vi "while_v0_v18.vi"() -> ()   [LabVIEW 2009]
panel:
  in  "Color Box":u32(colorbox)=16711695
  in  "X0":u16(slide)=73 scale=0.0..400.0
  in  "X1":u16(slide)=287 scale=0.0..400.0
  in  "Y1":u16(slide)=204 scale=300.0..0.0
  in  "Y0":u16(slide)=76 scale=300.0..0.0
  in  "stop":bool
  out "Picture":picture
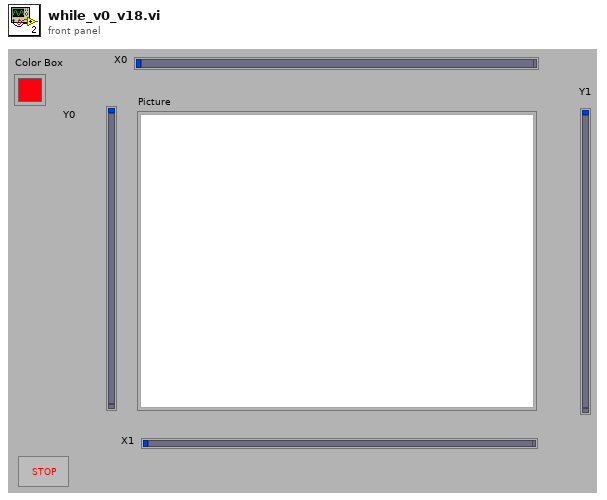
[diagram p1: front panel]
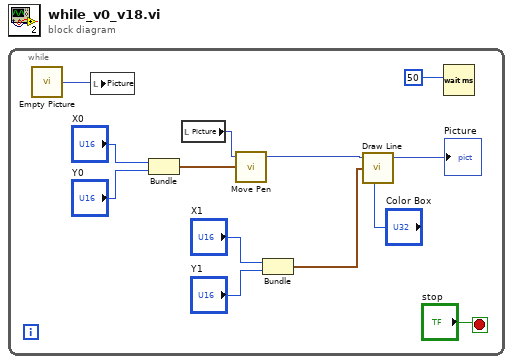
[diagram p0: block diagram]
diagram:
  n1 = while {
    stop <- "stop" stop-if-true
    n2 = call "Empty Picture"() -> ("empty picture"=w5:picture)
    n3 = local write "Picture"(w5) -> ()
    n4 = Bundle("X0"="X0", "Y0"="Y0") -> (w9:cluster{"X0":u16, "Y0":u16})  [unwired: 1 in]
    n5 = local read "Picture"() -> (w11:picture)
    n6 = call <vilib>:"Move Pen.vi"("new position"=w9, "picture"=w11) -> ("new picture"=w8:picture)  [unwired: 3 in]
    n7 = Bundle("X1"="X1", "Y1"="Y1") -> (w7:cluster{"X1":u16, "Y1":u16})  [unwired: 1 in]
    n8 = call <vilib>:"Draw Line.vi"("picture"=w8, "end point"=w7, "color(black)"="Color Box") -> ("new picture"=→"Picture":picture)  [unwired: 6 in]
    n9 = Wait (ms)(milliseconds to wait=50) -> ()  [unwired: 1 out]
  }
